vi "ReadLocationsNode.vi"(8 "Error In":errorcluster, 11 "Memory Node In":refnum<k20>) -> (0 "Error Out":errorcluster, 2 "Locations":string[](array[string]), 3 "Memory Node Out":refnum<k20>)   [LabVIEW 2012]
uses:
  <vilib>/xml/NI_XML.lvlib
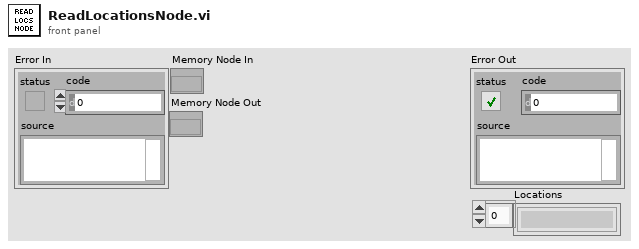
[diagram p1: front panel]
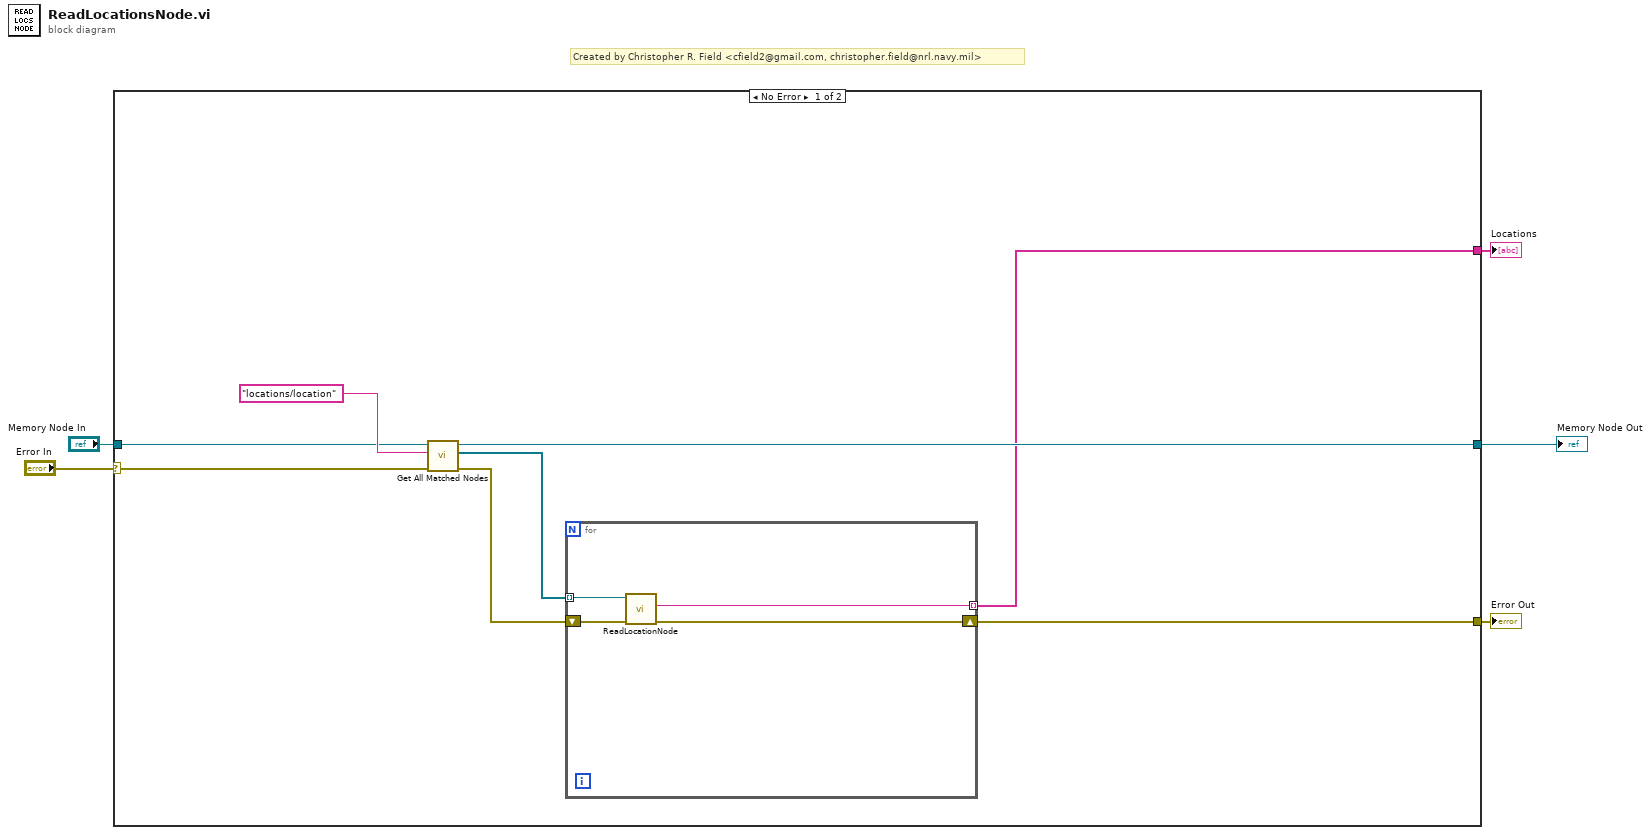
[diagram p0: block diagram]
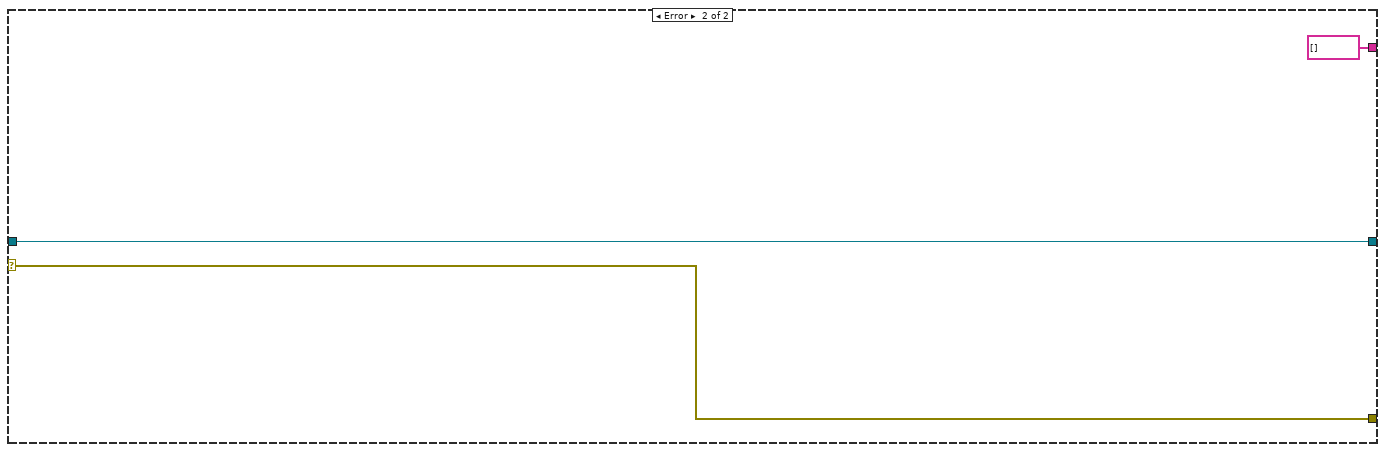
[diagram p2: hidden frame]
diagram:
  # "Created by Christopher R. Field <cfield2@gmail.com, christopher.field@nrl.navy.mil>"
  n1 = case shown="No Error" "Error In" {
    selector: "Error In" -> [w12 w19]
    tunnel: "Memory Node In" -> [w11 w20]
    tunnel: [w8 w20] -> w3
    tunnel: [w7 w19] -> w2
    tunnel: [w6 string[] []] -> w1
    frame No Error {
      n2 = call <vilib>:"Get All Matched Nodes.vi"("error in (no error)"=w12, "XPath expression"="locations/location", "node in"=w11) -> ("error out"=w9:errorcluster, "node result array"=w10:refnum<k20>[], "node out"=w8:refnum<k20>)  [unwired: 6 in]
      n3 = for {
        tunnel: w10 -> [w17] mode=indexing
        shift-right: [w15] -> w7
        shift-left: w9 -> [w16]
        tunnel: [w14] -> w6 mode=indexing
        n4 = call "ReadLocationNode.vi"("Error In"=w16, "Location Node In"=w17) -> ("Error Out"=w15:errorcluster, "Pattern"=w14:string)  [unwired: 7 in, 1 out]
      }
    }
    frame Error {
    }
  }
  "Memory Node Out" <- w3
  "Error Out" <- w2
  "Locations" <- w1
